vi "Interpolation (Control - Window Init Mem - LEO) Test.vi"() -> ()   [LabVIEW 2014]
uses:
  <vilib>/rvi/interface/nirviOpenFPGA/nirviOpenFPGA.xnode
  <vilib>/rvi/interface/nirviMethod/nirviMethod.xnode
  <vilib>/rvi/errors/niLvFpgaMergeErrorWithErrorCode.vi
  <vilib>/FPGAPlugInAG/Dynamic/niLvFpga_Run_Dynamic.vi
  <vilib>/FPGAPlugInAG/Dynamic/niLvFpga_Abort_Dynamic.vi
  <vilib>/rvi/interface/nirviCloseFPGA/nirviCloseFPGA.xnode
  <vilib>/rvi/interface/nirviReadWriteControl/nirviReadWriteControl.xnode
  FPGA Target/Test VIs/Double FFT Mesurament (Max Bin detection - Control - Windowing - LEO) test.vi
  NiFpgaLv.dll
  <vilib>/Utility/error.llb/Error Cluster From Error Code.vi
  <vilib>/rvi/interface/Simulation/niFpgaSimulationCallBeginRW.vi
  <vilib>/rvi/errors/niLvFpgaAdjustHostInterfaceError.vi
  <vilib>/FPGAPlugInAG/Dynamic/niLvFpga_ConfigureFifo_Dynamic.vi
  <vilib>/FPGAPlugInAG/Dynamic/niLvFpga_StartFifo_Dynamic.vi
  <vilib>/FPGAPlugInAG/Dynamic/niLvFpga_Close_Dynamic.vi
  <vilib>/platform/TimedLoop/XDataNode/XDataNode.xnode
  <vilib>/Platform/TimedLoop/XDataNode/nitl_modes.ctl
  <vilib>/Platform/TimedLoop/XDataNode/XDNodeRunTimeDep.lvlib
  <vilib>/Platform/TimedLoop/XDataNode/wakeup.ctl
  <vilib>/Platform/TimedLoop/XDataNode/timing_clust.ctl
panel:
  in  "Windowing":T1(ring)
  in  "first bin":i32=10
  in  "last bin":i32=255
  in  "lower limit 2":u32(slide)=677 scale=625.0..737.0
  in  "lower limit 1":u32(slide)=59 scale=0.0..112.0
  out "Detected Frequency Tone - (Hz)":dbl
  in  "stop":bool
  out "Max Bin":i32
  out "Max Amp":dbl format="%.2f"
  out "Prev Bin":i32
  out "Next Bin":i32
  out "Prev Amp":dbl format="%.2f"
  out "Next Amp":dbl format="%.2f"
  out "Interpolated Bin":dbl
  in  "Interpolation Method":T2(ring)=enum."Jain"
  # "ONLINE parameter"
  # "OFFLINE parameters"
  # "Max Detection FFT bin range"
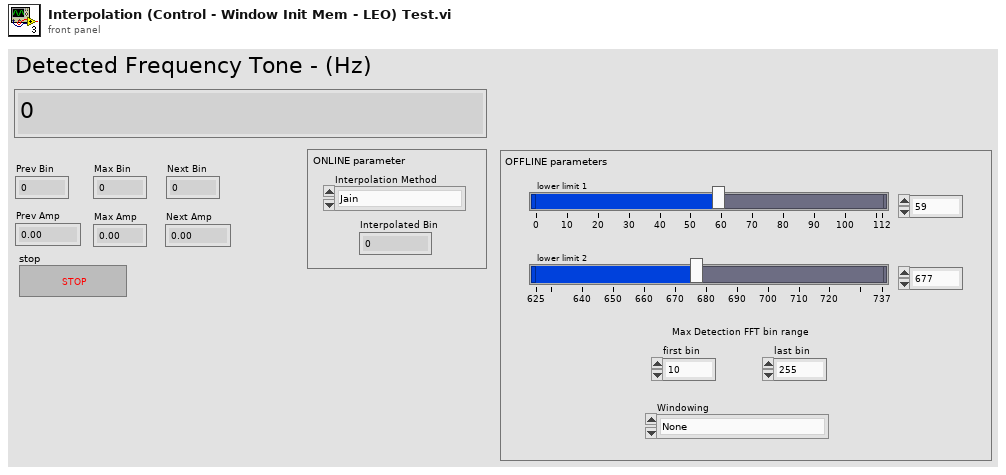
[diagram p1: front panel]
types:
  T1 = enum16{"None", "Hanning", "Hamming", "Blackman", "Blackman-Harris"}
  T2 = enum16{"Quadratic", "McLeodd", "Barycentric", "Jain"}
  T3 = typedef "XDNodeRunTimeDep.lvlib/timing_clust.ctl" = cluster{"Expected End [f-1]":u64, "Actual End [f-1]":u64, "Finished Late? [f-1]":bool, "Expected End [i-1]":u64, "Actual End [i-1]":u64, "Finished Late? [i-1]":bool, "Expected Start [i]":u64, "Actual Start [i]":u64, "Expected Start [f]":u64, "Actual Start [f]":u64, "Source Name":string, "Structure Name":string, "Period":i64, "Deadline":i64, "Offset":i64, "Start":i64, "Priority":i32, "Timeout":i32, "Mode":T4, "Wakeup Reason":T5, "Error":errorcluster, "Source Type":string, "Secondary Source Type":string, "Global End Time":u64, "Global Start Time":u64, "Frame Duration":u64, "Iteration Duration":u64, "Assigned CPU":i32, "I/O Scan Engine Mode":u32}
  T4 = typedef "XDNodeRunTimeDep.lvlib/nitl_modes.ctl" = enum32{"No Change", "Process missed periods, maintain original phase", "Discard missed periods, maintain original phase", "Process missed periods, ignore original phase", "Discard missed periods, ignore original phase"}
  T5 = typedef "XDNodeRunTimeDep.lvlib/wakeup.ctl" = enum32{"Normal", "Aborted", "Asynchronous wakeup", "Timing source error", "Timed loop error", "Timeout"}
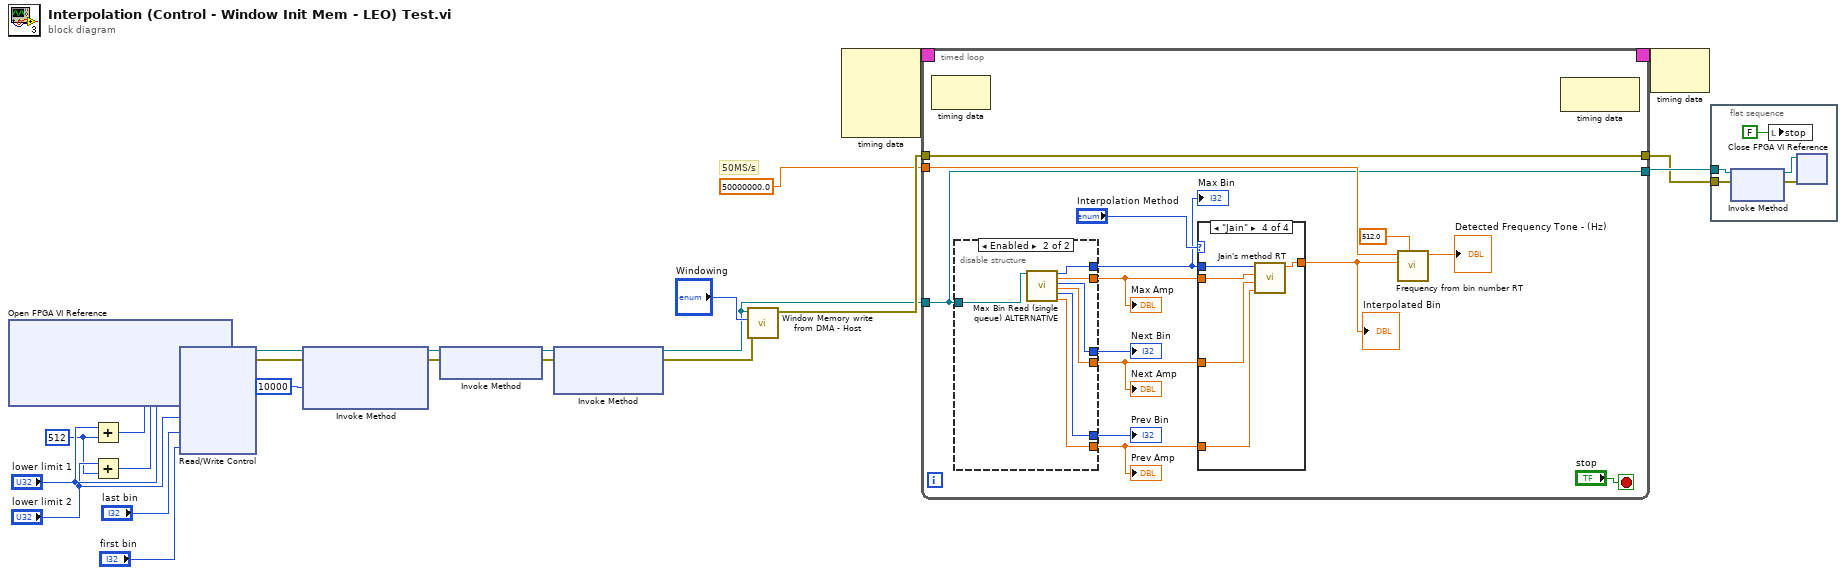
[diagram p0: block diagram]
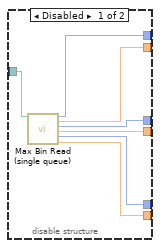
[diagram p2: hidden frame]
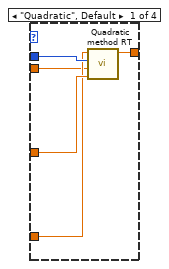
[diagram p3: hidden frame]
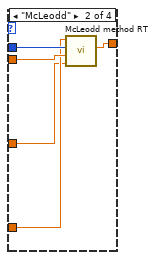
[diagram p4: hidden frame]
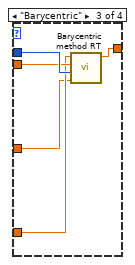
[diagram p5: hidden frame]
diagram:
  w19 = u32 512 ("y")
  # "50MS/s"
  n1 = xnode "Open FPGA VI Reference"() -> ("FPGA VI Reference Out"=w18:refnum<k20>, "error out"=w17:errorcluster)  [unwired: 2 in]
  n2 = Add(x="lower limit 1", y=w19) -> (x+y=w23:u32)
  n3 = Add(x="lower limit 2", y=w19) -> (x+y=w21:u32)
  n4 = xnode "Read/Write Control"("FPGA VI Reference In"=w18, "error in"=w17, "upper limit 1"=w23, "upper limit 2"=w21, "lower limit 1"="lower limit 1", "lower limit 2"="lower limit 2", "last bin"="last bin", "first bin"="first bin") -> ("FPGA VI Reference Out"=w11:refnum<k20>, "error out"=w10:errorcluster)
  n5 = xnode "Invoke Method"("FPGA VI Reference In"=w11, "error in"=w10, "Requested Depth"=u32 10000) -> ("FPGA VI Reference Out"=w9:refnum<k20>, "error out"=w8:errorcluster)  [unwired: 1 out]
  n6 = xnode "Invoke Method"("FPGA VI Reference In"=w9, "error in"=w8) -> ("FPGA VI Reference Out"=w6:refnum<k20>, "error out"=w7:errorcluster)
  n7 = xnode "Invoke Method"("FPGA VI Reference In"=w6, "error in"=w7) -> ("FPGA VI Reference Out"=w3:refnum<k20>, "error out"=w4:errorcluster)  [unwired: 1 in]
  n8 = call "Window Memory write from DMA - Host.vi"("error in"=w4, "Enum"="Windowing", "FPGA VI Reference In"=w3) -> ("error out"=w14:errorcluster)  [unwired: 5 in, 3 out]
  n9 = node-c288() -> (w2:T3)  [unwired: 4 in]
  n10 = timed-loop {
    tunnel: 50000000.0 ("Sample Rate (S/s)") -> [w38]
    tunnel: w14 -> [w37]
    tunnel: [w26] -> w16
    tunnel: [w37] -> w5
    tunnel: w3 -> [w26]
    timing: w2 -> [_]
    timing-out: [_] -> w1
    stop <- "stop" stop-if-true
    n11 = node-c288() -> ()  [unwired: 1 in, 1 out]
    n12 = disable-structure shown="Enabled" {
      disable-tunnel: [w48 w55] -> w33
      disable-tunnel: [w47 w54] -> w32
      disable-tunnel: [w46 w52] -> w31
      disable-tunnel: [w45 w50] -> w30
      disable-tunnel: [w44 w51] -> w29
      disable-tunnel: [w43 w53] -> w28
      disable-tunnel: w26 -> [w42 w49]
      frame Disabled {
        n13 = call "Max Bin Read (single queue).vi"("FPGA VI Reference In"=w42) -> ("Max Bin"=w48:i32, "Max Amp"=w47:dbl, "Next Bin"=w43:i32, "Next Amp"=w46:dbl, "Prev Bin"=w44:i32, "Prev Amp"=w45:dbl)  [unwired: 13 in]
      }
      frame Enabled {
        n14 = call "Max Bin Read (single queue) ALTERNATIVE.vi"("FPGA VI Reference In"=w49) -> ("Max Bin"=w55:i32, "Max Amp"=w54:dbl, "Next Bin"=w53:i32, "Next Amp"=w52:dbl, "Prev Bin"=w51:i32, "Prev Amp"=w50:dbl)  [unwired: 13 in]
      }
    }
    "Max Bin" <- w33
    "Max Amp" <- w32
    "Prev Bin" <- w29
    "Next Bin" <- w28
    "Prev Amp" <- w30
    "Next Amp" <- w31
    n15 = case shown="\"Jain\"" "Interpolation Method" {
      tunnel: w33 -> [w59 w64 w69 w74]
      tunnel: w32 -> [w56 w63 w68 w73]
      tunnel: w30 -> [w57 w62 w67 w72]
      tunnel: w31 -> [w58 w61 w66 w71]
      tunnel: [w60 w65 w70 w75] -> w34
      frame "Quadratic", Default {
        n16 = call "Quadratic method RT.vi"("Next Amplitude"=w58, "Max Amplitude"=w56, "Max bin"=w59, "Prev Amplitude"=w57) -> ("Bin"=w60:dbl)  [unwired: 7 in]
      }
      frame "McLeodd" {
        n17 = call "McLeodd method RT.vi"("Next Amp"=w61, "Max Amp"=w63, "Max Bin"=w64, "Prev Amp"=w62) -> ("Bin"=w65:dbl)  [unwired: 7 in]
      }
      frame "Barycentric" {
        n18 = call "Barycentric method RT.vi"("Next Amp"=w66, "Max Bin"=w69, "Max Amp"=w68, "Prev Amp"=w67) -> ("Bin"=w70:dbl)  [unwired: 7 in]
      }
      frame "Jain" {
        n19 = call "Jain's method RT.vi"("Prev Amp"=w72, "Next Amp"=w71, "Max Amp"=w73, "Max Bin"=w74) -> ("Bin"=w75:dbl)  [unwired: 7 in]
      }
    }
    "Interpolated Bin" <- w34
    n20 = call "Frequency from bin number RT.vi"("FFT size"=512.0, "Bin number"=w34, "Sample Rate (S/s)"=w38) -> ("Detected Frequency (Hz)"=→"Detected Frequency Tone - (Hz)":dbl)  [unwired: 8 in]
    n21 = node-c288() -> ()  [unwired: 1 in, 1 out]
  }
  n22 = node-c288(w1) -> ()  [unwired: 1 out]
  n23 = flat-sequence {
    tunnel: w16 -> [w78]
    tunnel: w5 -> [w77]
    frame #0 {
      n24 = xnode "Invoke Method"("FPGA VI Reference In"=w78, "error in"=w77) -> ("FPGA VI Reference Out"=w79:refnum<k20>, "error out"=w80:errorcluster)
      n25 = local write "stop"(FALSE ("stop")) -> ()
      n26 = xnode "Close FPGA VI Reference"("FPGA VI Reference In"=w79, "error in"=w80) -> ()  [unwired: 1 out]
    }
  }
